vi "st_str Global.vi"() -> ()   [LabVIEW 2017]
uses:
  controls/A5000_param.ctl
panel:
  in  "Tab Control":enum32{"Page 1", "Page 2", "A5000_param", "GUI"}(tab)
  out "WorkVoltmetr":bool
  out "WaitSignalGen":u32=100
  out "ChangeGenParam":bool
  in  "Frequency,kHz":dbl
  in  "UgenVrms":dbl
  out "GUICount":i32
  out "OscCount":i32
  out "meas":string[](array[string])=["10:51:54", "244.889E-3", "175.506E-3", "23.235E+0", "15.882E+0", "10 В", "10 В"]
  in  "StopCapCycle":bool
  out "detected_freq":dbl[](array[numeric]) format="%_4p"
  out "detected_amp":dbl[](array[numeric]) format="%_5p"
  out "Osc":waveform(dbl)[](array[waveform])
  out "OscCon":bool
  in  "About_prg":T1={"Версия:"="1.0", "Наименование ПО:"="voltmetr.exe", "Год выпуска:"="2026", "Производитель:"="ООО \"НПП Датчик\"", "MD5"="", "Наименование ПО полное:"="Вольтметр", "Build"="1.0.0"}
  in  "A5000_param":T2={"ChannelA"={"Enabled"=FALSE, "Coupling"=1, "Range"=6, "Analogue Offset"=0.0}, "ChannelB"={"Enabled"=FALSE, "Coupling"=1, "Range"=6, "Analogue Offset"=0.0}, "Trigger"={"Trigger Enabled"=FALSE, "Trigger Source"=enum."Channel A", "Trigger Threshold (volts)"=0.0, "Trigger Direction"=2, "Trigger Delay (samples)"=0, "Auto Trigger Time (ms)"=1000}, "MaxADCvalue"=0, "handle"=0, "Acquisition"={"preTriggerSamples"=0, "postTriggerSamples"=12500000, "timebase"=4, "Down-Sample Mode"=2, "Down Sample Ratio"=10}, "Device Info"={"Driver Version"="", "USB Version"="", "Hardware"="", "Variant"="", "Batch and Serial"="", "Cal Date"="", "Kernel Version"="", "Digital HW Version"="", "Analogue HW Version"="", "MSO"=FALSE, "Number of channels"=0}, "Properties"={"Sample Frequency"=0.0, "Sample Rate"=0.0, "Max Samples Available"=0, "Number of Samples"=0, "Total Capture Time (sec) "=0.0, "Max Total Capture Time Available (sec)"=0.0}, "Resolution"=3, "EmulateV"=FALSE, "General AWG Settings"={"Peak-to-Peak Voltage (microvolts)"=2000000, "Offset Voltage (microvolts)"=0, "Wave Type"=0, "Sweep Type"=0, "Shots"=0, "Sweeps"=0, "Trigger Type"=0, "Trigger Source"=0, "Ext. Threshold (ADC count)"=0, "White Noise/PRBS"=0}, "Standard Waveform Settings"={"Start Frequency"=1000.0, "Stop Frequency"=1000.0, "Increment"=0.0, "Dwell Time (seconds)"=0.0}, "Arbitrary Waveform Settings"={"Arbirary waveform file path"=path "", "Index Mode"=0}, "AutoDiapChA"=FALSE, "AutoDiapChB"=FALSE} {"Arbitrary Waveform Settings"."Index Mode" items=["Single", "Dual", "Quad"]; "Standard Waveform Settings"."Stop Frequency" min=0.03 max=1000000.0; "Standard Waveform Settings"."Start Frequency" min=0.03 max=1000000.0; "General AWG Settings"."White Noise/PRBS" items=["Normal", "White Noise", "PRBS"]; "General AWG Settings"."Trigger Source" items=["None", "Scope Trigger", "Aux. In", "Ext. In", "Software Trigger"]; "General AWG Settings"."Trigger Type" items=["Rising", "Falling", "Gate High", "Gate Low"]; "General AWG Settings"."Sweep Type" items=["Up", "Down", "Up-Down", "Down-Up"]; "General AWG Settings"."Wave Type" items=["Sine", "Square", "Triangle", "Ramp Up", "Ramp Down", "Sinc", "Gaussian", "Half Sine", "DC", "Arbitrary"]; "Resolution" items=["8-bit", "12-bit", "14-bit", "15-bit (max. 2 ch.)", "16-bit (max. 1 ch.)"]; "Properties"."Max Total Capture Time Available (sec)" format="%.3p"; "Properties"."Sample Frequency" format="%.3p"; "Properties"."Sample Rate" format="%.3p"; "Properties"."Max Samples Available" format="%.3p"; "Properties"."Total Capture Time (sec)" format="%.3p"; "Acquisition"."Down Sample Ratio" min=1 step=1; "Acquisition"."Down-Sample Mode" items=["None"=0, "Aggregate"=1, "Decimate"=2, "Average"=4]; "Trigger"."Trigger Direction" items=["Rising"=2, "Falling"=3]; "ChannelB"."Range" items=["10 mV", "20 mV", "50 mV", "100 mV", "200 mV", "500 mV", "1 V", "2 V", "5 V", "10 V", "20 V"]; "ChannelB"."Coupling" items=["AC", "DC"]; "ChannelA"."Range" items=["10 mV", "20 mV", "50 mV", "100 mV", "200 mV", "500 mV", "1 V", "2 V", "5 V", "10 V", "20 V"]; "ChannelA"."Coupling" items=["AC", "DC"]}
  out "GUI_Gen":refnum<vi>[](array[refnum])
  out "GUI_Spectrogramm":refnum<vi>[](array[refnum])
  out "GUI_Waveform":refnum<vi>[](array[refnum])
  out "GUI_Voltmetr":refnum<vi>[](array[refnum])
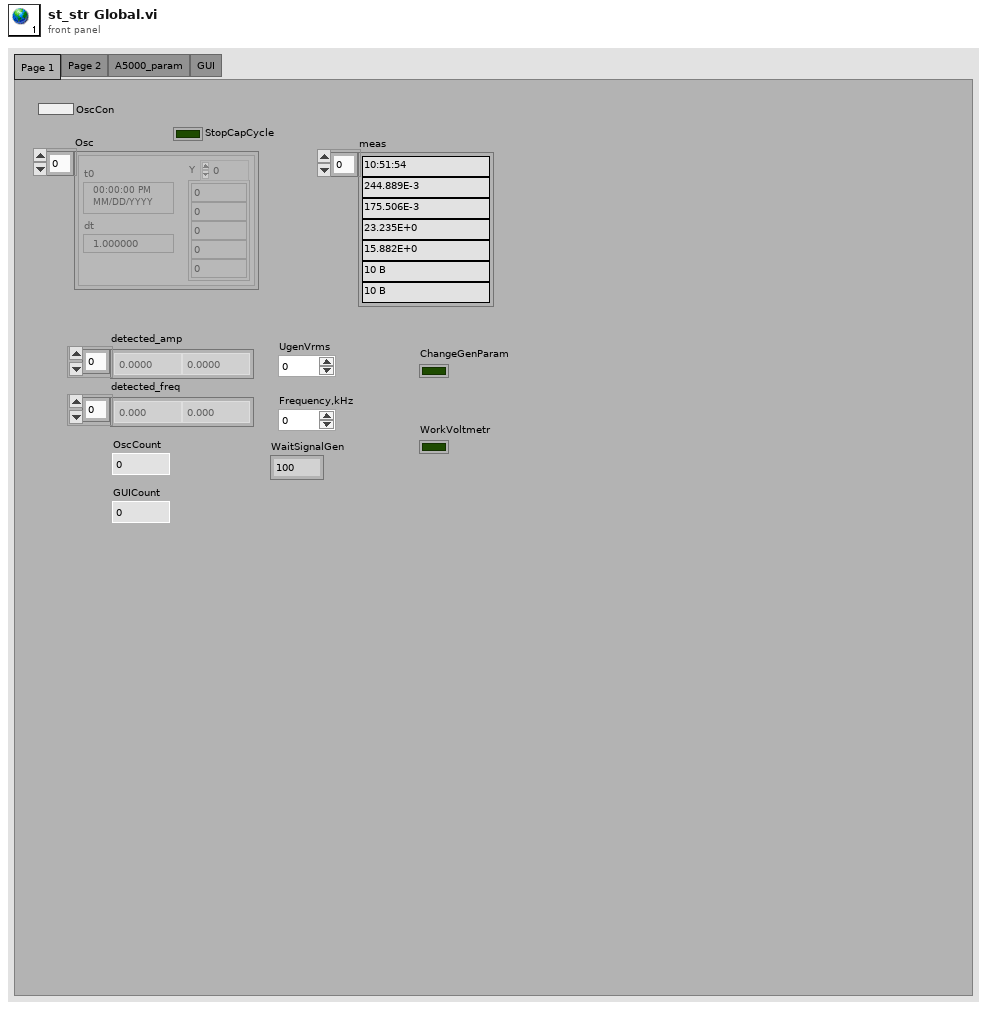
[diagram p1: front panel]
types:
  T1 = cluster{"Версия:":string, "Наименование ПО:":string, "Год выпуска:":string, "Производитель:":string, "MD5":string, "Наименование ПО полное:":string, "Build":string}
  T2 = typedef "A5000_param.ctl" = cluster{"ChannelA":cluster{"Enabled":bool, "Coupling":i16, "Range":u16, "Analogue Offset":sgl}, "ChannelB":cluster{"Enabled":bool, "Coupling":i16, "Range":u16, "Analogue Offset":sgl}, "Trigger":cluster{"Trigger Enabled":bool, "Trigger Source":enum16{"Channel A", "Channel B", "Channel C", "Channel D", "Ext."}, "Trigger Threshold (volts)":dbl, "Trigger Direction":u16, "Trigger Delay (samples)":u32, "Auto Trigger Time (ms)":i16}, "MaxADCvalue":i16, "handle":i16, "Acquisition":cluster{"preTriggerSamples":i32, "postTriggerSamples":i32, "timebase":u32, "Down-Sample Mode":u32, "Down Sample Ratio":u32}, "Device Info":cluster{"Driver Version":string, "USB Version":string, "Hardware":string, "Variant":string, "Batch and Serial":string, "Cal Date":string, "Kernel Version":string, "Digital HW Version":string, "Analogue HW Version":string, "MSO":bool, "Number of channels":i16}, "Properties":cluster{"Sample Frequency":sgl, "Sample Rate":sgl, "Max Samples Available":i32, "Number of Samples":u32, "Total Capture Time (sec) ":sgl, "Max Total Capture Time Available (sec)":sgl}, "Resolution":i32, "EmulateV":bool, "General AWG Settings":cluster{"Peak-to-Peak Voltage (microvolts)":u32, "Offset Voltage (microvolts)":i32, "Wave Type":u32, "Sweep Type":u32, "Shots":u32, "Sweeps":u32, "Trigger Type":u32, "Trigger Source":u32, "Ext. Threshold (ADC count)":i16, "White Noise/PRBS":u32}, "Standard Waveform Settings":cluster{"Start Frequency":dbl, "Stop Frequency":dbl, "Increment":dbl, "Dwell Time (seconds)":dbl}, "Arbitrary Waveform Settings":cluster{"Arbirary waveform file path":path, "Index Mode":u32}, "AutoDiapChA":bool, "AutoDiapChB":bool}
diagram:
